vi "Save JPEG2000.vi"(6 "compression":i32=500, 8 "error in (no error)":errorcluster, 10 "File Path":path, 11 "Image in":T1) -> (0 "error out":errorcluster, 3 "Image out (dup)":T1)   [LabVIEW 2026]
uses:
  <vilib>/vision/Image Controls.llb/IMAQ Image.ctl
  target/release/jpeg2000_export.dll
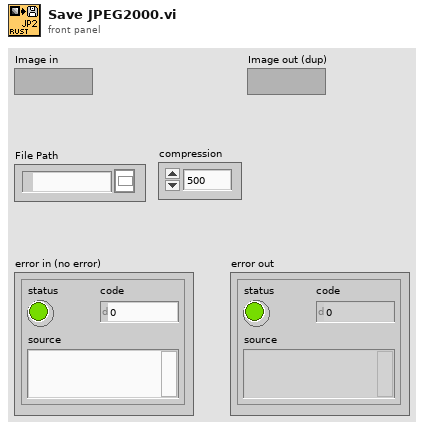
[diagram p1: front panel]
types:
  T1 = typedef "IMAQ Image.ctl" = refnum<image>
  T2 = enum32{"Map Pixel Pointer", "Unmap Pixel Pointer", "Get Pixels Infos"}
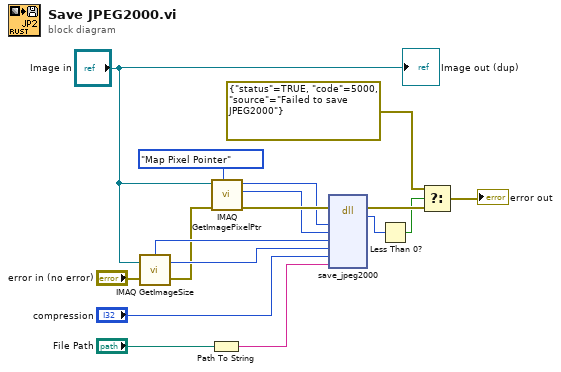
[diagram p0: block diagram]
diagram:
  n1 = call "IMAQ GetImageSize"("Image"="Image in", "error in (no error)"="error in (no error)") -> ("Y Resolution"=w8:i32, "X Resolution"=w7:i32, "error out"=w1:errorcluster)  [unwired: 2 in]
  n2 = Path To String(path="File Path") -> (string=w11:string)
  n3 = call "IMAQ GetImagePixelPtr"("Function"=T2."Map Pixel Pointer", "error in (no error)"=w1, "Image"="Image in") -> ("error out"=w12:errorcluster, "LineWidth(Pixels)"=w9:i32, "Pixel Pointer out"=w5:u64)  [unwired: 3 in, 3 out]
  n4 = dll-call lib="C:/Users/108003658/Desktop/r-lv-jpeg2000/target/release/jpeg2000_export.dll" fn="save_jpeg2000"(error in=w12, "ptr"=w5, "stride"=w9, "width"=w7, "height"=w8, "compression"="compression", "path"=w11) -> (error out=w16:errorcluster, "return type"=w13:i32)  [unwired: 8 in, 1 out]
  n5 = Less Than 0?(x=w13) -> (x < 0?=w14:bool)
  n6 = Select(t=errorcluster {"status"=TRUE, "code"=5000, "source"="Failed to save JPEG2000"} ("error out"), s=w14, f=w16) -> (s? t:f=→"error out":errorcluster)
  "Image out (dup)" <- "Image in"
